vi "WaitForNextReadTriggerTime.vi"(8 "Error In":errorcluster, 10 "RPM Update Data":T6, 11 "MasterCluster In":T1={"Plate Reader State"=enum."Idle", "SMPAutomationClientRef"=refnum, "CommandCompleted Refnum"=refnum, "InstrumentStatusChanged Refnum"=refnum, "ErrorReport Refnum"=refnum, "Read Start Time"=timestamp(0 s since 1904-01-01), "Read Count"=0, "Active Column"=0, "Raw Result"="", "GetDataCopy CMD Queue ID"=0, "Error Log"="", "Column Data"={"Col Absorbances"=[], "Col Read Times"=[], "Col Read Positions (deg)"=[], "Temperature (degC)"=0.0, "Active Column"=0, "Previous Column"=0, "Column Read Start Time"=timestamp(0 s since 1904-01-01), "Column Busy Start Time"=timestamp(0 s since 1904-01-01), "Column Busy Stop Time"=timestamp(0 s since 1904-01-01), "Column Mark Read Start Time"=timestamp(0 s since 1904-01-01), "Column Mark Read Stop Time"=timestamp(0 s since 1904-01-01)}, "Grid"=[[0.0, 0.0, 0.0, 0.0, 0.0, 0.0, 0.0, 0.0, 0.0, 0.0, 0.0, 0.0], [0.0, 0.0, 0.0, 0.0, 0.0, 0.0, 0.0, 0.0, 0.0, 0.0, 0.0, 0.0], [0.0, 0.0, 0.0, 0.0, 0.0, 0.0, 0.0, 0.0, 0.0, 0.0, 0.0, 0.0], [0.0, 0.0, 0.0, 0.0, 0.0, 0.0, 0.0, 0.0, 0.0, 0.0, 0.0, 0.0], [0.0, 0.0, 0.0, 0.0, 0.0, 0.0, 0.0, 0.0, 0.0, 0.0, 0.0, 0.0], [0.0, 0.0, 0.0, 0.0, 0.0, 0.0, 0.0, 0.0, 0.0, 0.0, 0.0, 0.0], [0.0, 0.0, 0.0, 0.0, 0.0, 0.0, 0.0, 0.0, 0.0, 0.0, 0.0, 0.0], [0.0, 0.0, 0.0, 0.0, 0.0, 0.0, 0.0, 0.0, 0.0, 0.0, 0.0, 0.0]], "Column Read Start Time"=timestamp(0 s since 1904-01-01), "Previous Column"=0, "Raw Log File Refnum"=refnum, "Read Specifications"={"Read Period (min)"=0.0, "Experiment Duration (min)"=0.0, "Number of Columns"=0, "Apex Deviance (deg)"=0.0, "Log File Name"="", "Number of Wavelengths"=0, "Timing Profile"=enum."No Timing", "Column Switch Delay"=0.0, "Column Repeat Delay"=0.0, "Audible Read Delay"=0.0, "Audible Read Interval"=0.0, "SMP Protocol Path"=path "", "Upper Busy Delay Limit"=inf, "Lower Busy Delay Limit"=-inf, "Upper Busy Interval Limit"=inf, "Lower Busy Interval Limit"=-inf, "Number of Rows"=0, "Plate Reader COM Port"=""}, "Plate Reader Crash State"=enum."Idle", "Consecutive Missed Reads"=0, "Excel File Refnum"=refnum} {"Column Data"."Column Mark Read Stop Time" format="%<%H:%M:%S%3u\n%x>T"; "Column Data"."Column Mark Read Start Time" format="%<%H:%M:%S%3u\n%x>T"; "Column Data"."Column Busy Stop Time" format="%<%H:%M:%S%3u\n%x>T"; "Column Data"."Column Busy Start Time" format="%<%H:%M:%S%3u\n%x>T"; "Column Data"."Column Read Start Time" format="%<%H:%M:%S%3u\n%x>T"; "Column Data"."Col Read Times" format="%<%H:%M:%S%3u\n%x>T"}) -> (0 "Error Out":errorcluster, 2 "Time Waited (ms)":dbl, 3 "MasterCluster Out":T1={"Plate Reader State"=enum."Idle", "SMPAutomationClientRef"=refnum, "CommandCompleted Refnum"=refnum, "InstrumentStatusChanged Refnum"=refnum, "ErrorReport Refnum"=refnum, "Read Start Time"=timestamp(0 s since 1904-01-01), "Read Count"=0, "Active Column"=0, "Raw Result"="", "GetDataCopy CMD Queue ID"=0, "Error Log"="", "Column Data"={"Col Absorbances"=[], "Col Read Times"=[], "Col Read Positions (deg)"=[], "Temperature (degC)"=0.0, "Active Column"=0, "Previous Column"=0, "Column Read Start Time"=timestamp(0 s since 1904-01-01), "Column Busy Start Time"=timestamp(0 s since 1904-01-01), "Column Busy Stop Time"=timestamp(0 s since 1904-01-01), "Column Mark Read Start Time"=timestamp(0 s since 1904-01-01), "Column Mark Read Stop Time"=timestamp(0 s since 1904-01-01)}, "Grid"=[[0.0, 0.0, 0.0, 0.0, 0.0, 0.0, 0.0, 0.0, 0.0, 0.0, 0.0, 0.0], [0.0, 0.0, 0.0, 0.0, 0.0, 0.0, 0.0, 0.0, 0.0, 0.0, 0.0, 0.0], [0.0, 0.0, 0.0, 0.0, 0.0, 0.0, 0.0, 0.0, 0.0, 0.0, 0.0, 0.0], [0.0, 0.0, 0.0, 0.0, 0.0, 0.0, 0.0, 0.0, 0.0, 0.0, 0.0, 0.0], [0.0, 0.0, 0.0, 0.0, 0.0, 0.0, 0.0, 0.0, 0.0, 0.0, 0.0, 0.0], [0.0, 0.0, 0.0, 0.0, 0.0, 0.0, 0.0, 0.0, 0.0, 0.0, 0.0, 0.0], [0.0, 0.0, 0.0, 0.0, 0.0, 0.0, 0.0, 0.0, 0.0, 0.0, 0.0, 0.0], [0.0, 0.0, 0.0, 0.0, 0.0, 0.0, 0.0, 0.0, 0.0, 0.0, 0.0, 0.0]], "Column Read Start Time"=timestamp(0 s since 1904-01-01), "Previous Column"=0, "Raw Log File Refnum"=refnum, "Read Specifications"={"Read Period (min)"=0.0, "Experiment Duration (min)"=0.0, "Number of Columns"=0, "Apex Deviance (deg)"=0.0, "Log File Name"="", "Number of Wavelengths"=0, "Timing Profile"=enum."No Timing", "Column Switch Delay"=0.0, "Column Repeat Delay"=0.0, "Audible Read Delay"=0.0, "Audible Read Interval"=0.0, "SMP Protocol Path"=path "", "Upper Busy Delay Limit"=inf, "Lower Busy Delay Limit"=-inf, "Upper Busy Interval Limit"=inf, "Lower Busy Interval Limit"=-inf, "Number of Rows"=0, "Plate Reader COM Port"=""}, "Plate Reader Crash State"=enum."Idle", "Consecutive Missed Reads"=0, "Excel File Refnum"=refnum} {"Column Data"."Column Mark Read Stop Time" format="%<%H:%M:%S%3u\n%x>T"; "Column Data"."Column Mark Read Start Time" format="%<%H:%M:%S%3u\n%x>T"; "Column Data"."Column Busy Stop Time" format="%<%H:%M:%S%3u\n%x>T"; "Column Data"."Column Busy Start Time" format="%<%H:%M:%S%3u\n%x>T"; "Column Data"."Column Read Start Time" format="%<%H:%M:%S%3u\n%x>T"; "Column Data"."Col Read Times" format="%<%H:%M:%S%3u\n%x>T"})   [LabVIEW 2014]
uses:
  RPMUpdateData.ctl
  MasterCluster.ctl
  PlateReaderState.ctl
  C:/Program Files (x86)/Molecular Devices/SoftMax Pro 6.5.1 Automation SDK/SoftMaxPro.AutomationClient.dll
  Program Files (x86)/Molecular Devices/SoftMax Pro 6.5.1 Automation SDK/SoftMaxPro.AutomationClient.dll
  ColumnData.ctl
  ReadSpecifications.ctl
  TimingProfile.ctl
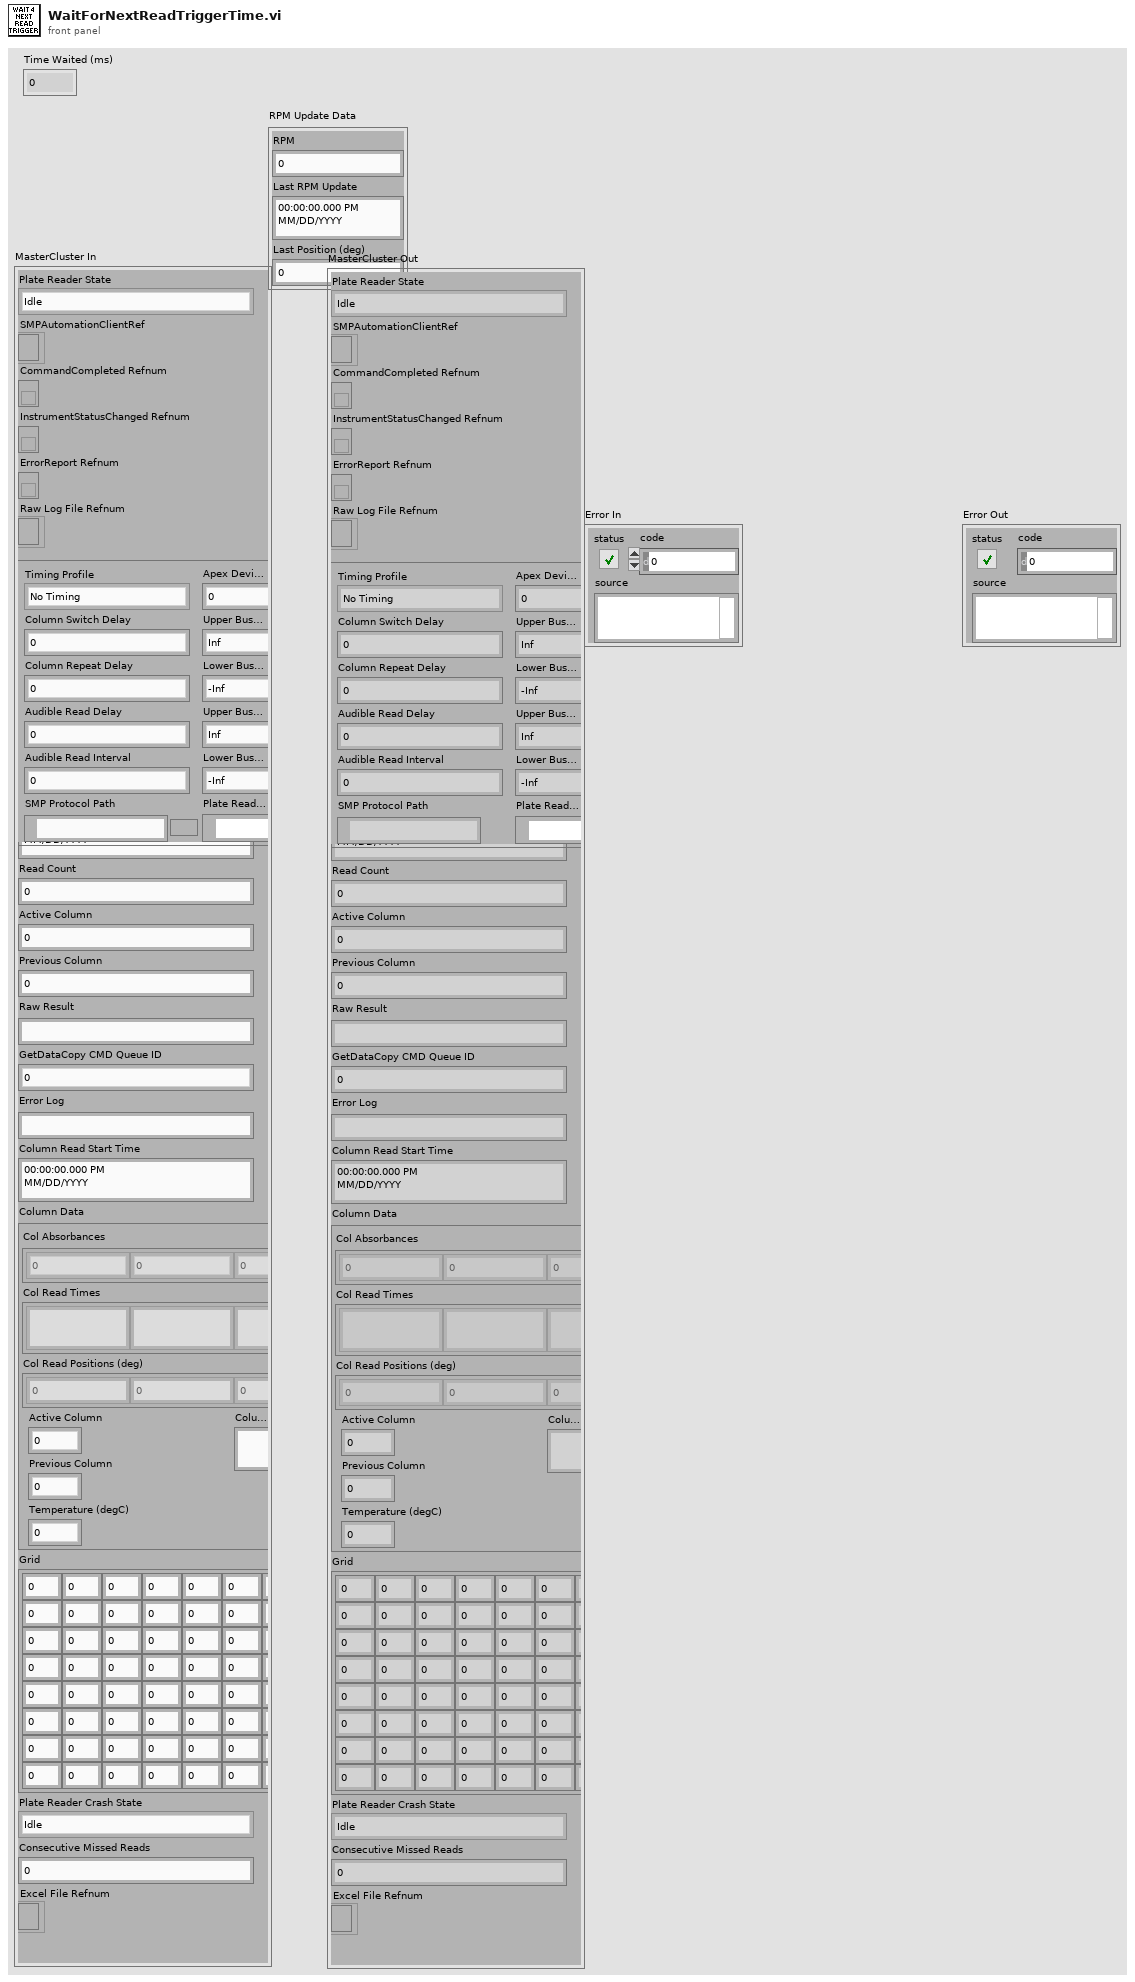
[diagram p1: front panel]
types:
  T1 = typedef "MasterCluster.ctl" = cluster{"Plate Reader State":T2, "SMPAutomationClientRef":refnum<k24>, "CommandCompleted Refnum":refnum<k27>, "InstrumentStatusChanged Refnum":refnum<k27>, "ErrorReport Refnum":refnum<k27>, "Read Start Time":timestamp, "Read Count":u64, "Active Column":u64, "Raw Result":string, "GetDataCopy CMD Queue ID":i32, "Error Log":string, "Column Data":T3, "Grid":dbl[][], "Column Read Start Time":timestamp, "Previous Column":u64, "Raw Log File Refnum":refnum<file>, "Read Specifications":T4, "Plate Reader Crash State":T2, "Consecutive Missed Reads":u64, "Excel File Refnum":refnum<file>}
  T2 = typedef "PlateReaderState.ctl" = enum16{"Idle", "Run", "Wait", "Read", "Init", "Exit", "Stop"}
  T3 = typedef "ColumnData.ctl" = cluster{"Col Absorbances":dbl[], "Col Read Times":timestamp[], "Col Read Positions (deg)":dbl[], "Temperature (degC)":dbl, "Active Column":u64, "Previous Column":u64, "Column Read Start Time":timestamp, "Column Busy Start Time":timestamp, "Column Busy Stop Time":timestamp, "Column Mark Read Start Time":timestamp, "Column Mark Read Stop Time":timestamp}
  T4 = typedef "ReadSpecifications.ctl" = cluster{"Read Period (min)":dbl, "Experiment Duration (min)":dbl, "Number of Columns":u64, "Apex Deviance (deg)":dbl, "Log File Name":string, "Number of Wavelengths":u64, "Timing Profile":T5, "Column Switch Delay":dbl, "Column Repeat Delay":dbl, "Audible Read Delay":dbl, "Audible Read Interval":dbl, "SMP Protocol Path":path, "Upper Busy Delay Limit":dbl, "Lower Busy Delay Limit":dbl, "Upper Busy Interval Limit":dbl, "Lower Busy Interval Limit":dbl, "Number of Rows":u64, "Plate Reader COM Port":refnum<visa-resource-name>}
  T5 = typedef "TimingProfile.ctl" = enum16{"No Timing", "24-Well Fluorescence", "48-Well Fluorescence", "96-Well Fluorescence", "96-Well Absorbance", "Custom Timing"}
  T6 = typedef "RPMUpdateData.ctl" = cluster{"RPM":dbl, "Last RPM Update":timestamp, "Last Position (deg)":dbl}
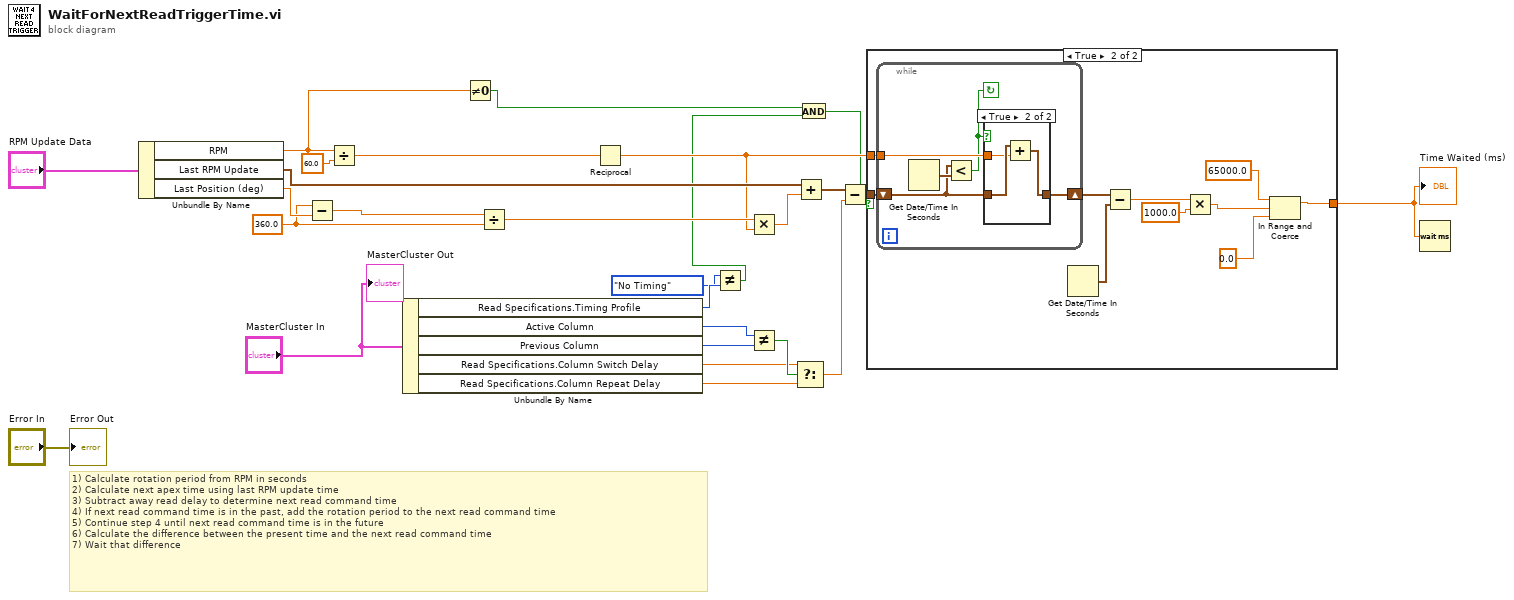
[diagram p0: block diagram]
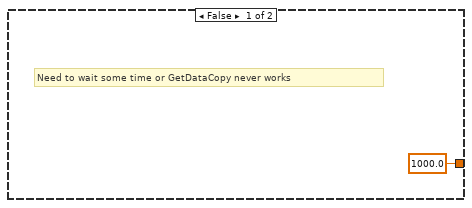
[diagram p2: hidden frame]
diagram:
  w12 = 360.0
  # "1) Calculate rotation period from RPM in seconds\n2) Calculate next apex time using last RPM update time\n3) Subtract away read delay to determine next read command time\n4) If next read command time is in the past, add the rotation period to the next read command time\n5) Continue step 4 until next read command time is in the future\n6) Calculate the difference between the present time and the next read command time\n7) Wait that difference"
  n1 = Unbundle By Name("RPM Update Data") -> ("RPM"=w6:dbl, "Last RPM Update"=w22:timestamp, "Last Position (deg)"=w14:dbl)
  n2 = Subtract(x=w12, y=w14) -> (x-y=w13:dbl)
  n3 = Divide(x=w6, y=60.0) -> (x/y=w26:dbl)
  n4 = Unbundle By Name("MasterCluster In") -> ("Read Specifications.Timing Profile"=w5:T5, "Active Column"=w17:u64, "Previous Column"=w16:u64, "Read Specifications.Column Switch Delay"=w10:dbl, "Read Specifications.Column Repeat Delay"=w9:dbl)
  n5 = Not Equal To 0?(x=w6) -> (x != 0?=w3:bool)
  n6 = Divide(x=w13, y=w12) -> (x/y=w20:dbl)
  n7 = Reciprocal(x=w26) -> (1/x=w19:dbl)
  n8 = Not Equal?(x=TimingProfile."No Timing" ("y"), y=w5) -> (x != y?=w2:bool)
  n9 = Multiply(x=w20, y=w19) -> (x*y=w18:dbl)
  n10 = Not Equal?(x=w17, y=w16) -> (x != y?=w11:bool)
  n11 = Select(t=w10, s=w11, f=w9) -> (s? t:f=w8:dbl)
  n12 = Add(x=w22, y=w18) -> (x+y=w25:timestamp)
  n13 = And(x=w3, y=w2) -> (x .and. y?=w1:bool)
  n14 = Subtract(x=w25, y=w8) -> (x-y=w24:timestamp)
  n15 = case shown="True" w1 {
    tunnel: w24 -> [_ w38]
    tunnel: w19 -> [_ w33]
    tunnel: [1000.0 ("upper limit") w29] -> w7
    frame False {
      # "Need to wait some time or GetDataCopy never works"
    }
    frame True {
      n16 = while {
        tunnel: w33 -> [w41]
        shift-right: [w40] -> w35
        shift-left: w38 -> [w42]
        stop <- w39 continue-if-true
        n17 = Get Date/Time In Seconds() -> (seconds since 1Jan1904=w43:timestamp)
        n18 = Less?(x=w42, y=w43) -> (x < y?=w39:bool)
        n19 = case shown="True" w39 {
          tunnel: w42 -> [w44 w47]
          tunnel: w41 -> [_ w46]
          tunnel: [w44 w45] -> w40
          frame False {
          }
          frame True {
            n20 = Add(x=w47, y=w46) -> (x+y=w45:timestamp)
          }
        }
      }
      n21 = Get Date/Time In Seconds() -> (seconds since 1Jan1904=w34:timestamp)
      n22 = Subtract(x=w35, y=w34) -> (x-y=w37:dbl)
      n23 = Multiply(x=w37, y=1000.0) -> (x*y=w32:dbl)
      n24 = In Range and Coerce(upper limit=65000.0, x=w32, lower limit=0.0) -> (coerced(x)=w29:dbl)  [unwired: 1 out]
    }
  }
  "Time Waited (ms)" <- w7
  n25 = Wait (ms)(milliseconds to wait=w7) -> ()  [unwired: 1 out]
  "Error Out" <- "Error In"
  "MasterCluster Out" <- "MasterCluster In"
